vi "Batch_ID_Generator (SubVI).vi"() -> (3 "String":string)   [LabVIEW 2019]
uses:
  <vilib>/numeric/Random Number (Range) U64.vi
  <vilib>/numeric/sub_Random U32.vi
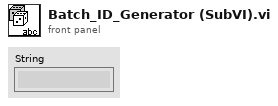
[diagram p1: front panel]
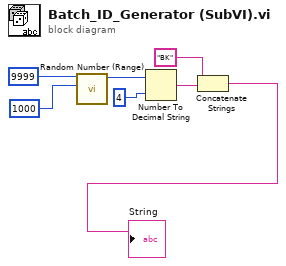
[diagram p0: block diagram]
diagram:
  n1 = call-poly <vilib>:"Random Number (Range).vi"("lower bound (0)"=u64 1000, "upper bound (100)"=u64 9999) -> ("number"=w3:u64)  [unwired: 9 in]
  n2 = Number To Decimal String(number=w3, width (-)=i16 4) -> (decimal integer string=w6:string)
  n3 = Concatenate Strings("BK" ("string"), w6) -> (→"String":string)
